vi "Get Column I64.vi"(8 "error in (no error)":errorcluster, 11 "PQ Result  in":refnum<class "PQ Result.lvclass">) -> (0 "error out":errorcluster, 2 "DBL":i64, 3 "PQ Result  out":refnum<class "PQ Result.lvclass">)   [LabVIEW 2013, in "PQ Result.lvclass"]
uses:
  PQ Result.lvclass
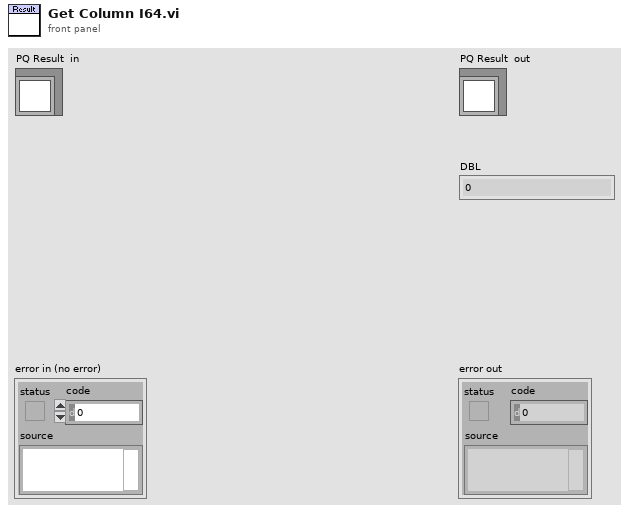
[diagram p1: front panel]
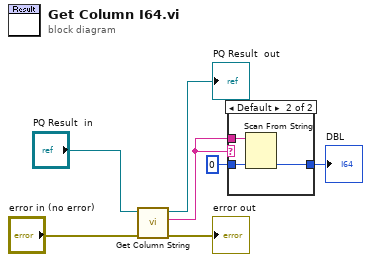
[diagram p0: block diagram]
diagram:
  n1 = call "Get Column String.vi"("error in (no error)"="error in (no error)", "PQ Result  in"="PQ Result  in") -> ("error out"=→"error out":errorcluster, "String"=w2:string, "PQ Result  out"=→"PQ Result  out":refnum<class "PQ Result.lvclass">)  [unwired: 7 in]
  n2 = case shown="Default" w2 {
    tunnel: w2 -> [_ w11]
    tunnel: [w8 w10] -> w3
    tunnel: i64 0 -> [w8 w9]
    frame "" {
    }
    frame Default {
      n3 = Scan From String(input string=w11, default 1=w9) -> (output 1=w10:i64)  [unwired: 3 in, 3 out]
    }
  }
  "DBL" <- w3
